vi "Defect detection.vi"(7 "File Path":path=path "C:/BeamViewImage/TESTIMAGE.png", 8 "error in":errorcluster, 10 "ROI Descriptors (Quantify 1)":T1(array[cluster])=[{"Global Rectangle"=[0, 0, 1280, 1024], "Contours"=[{"ID"=enum."External", "Type"=3, "Coordinates"=[0, 0, 1280, 1024]}]}] {"Contours"."Type" items=["No Selection", "Point", "Line", "Rectangle", "Oval", "Polygon", "Freehand Region", "Annulus", "Unused2", "Unused3", "Broken Line", "Freehand Line", "Rotated Rectangle"]}, 11 "Method (Filters 1)":T2(ring)=enum."Sobel") -> (0 "error out":errorcluster, 3 "Standard Variation":sgl)   [LabVIEW 2018]
uses:
  <vilib>/vision/NI_Vision_Development_Module.lvlib
panel:
  out "Image Out":T3(plugin-control)
  out "Results (Quantify 1)":sgl[][](array[numeric]) format="%.2f"
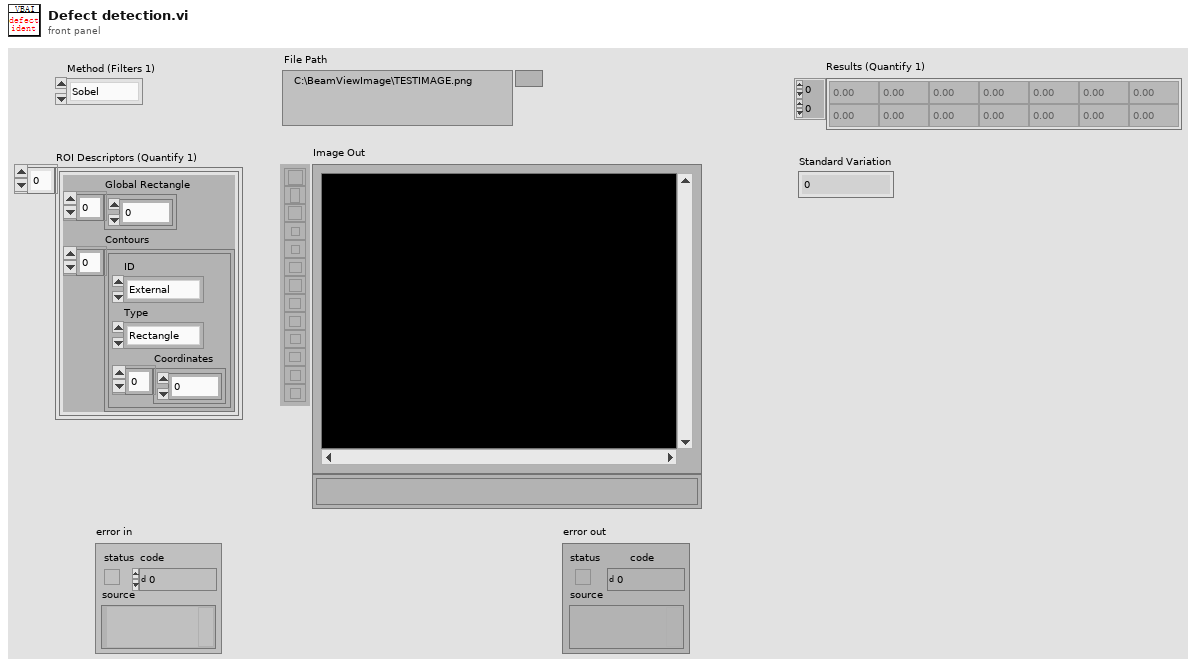
[diagram p1: front panel]
types:
  T1 = cluster{"Global Rectangle":i32[], "Contours":cluster{"ID":enum32{"External", "Internal"}, "Type":u32, "Coordinates":i32[]}[]}[]
  T2 = enum32{"Differentiation", "Gradient", "Prewitt", "Roberts", "Sigma", "Sobel"}
  T3 = typedef "IMAQ Image.ctl" = refnum<image>
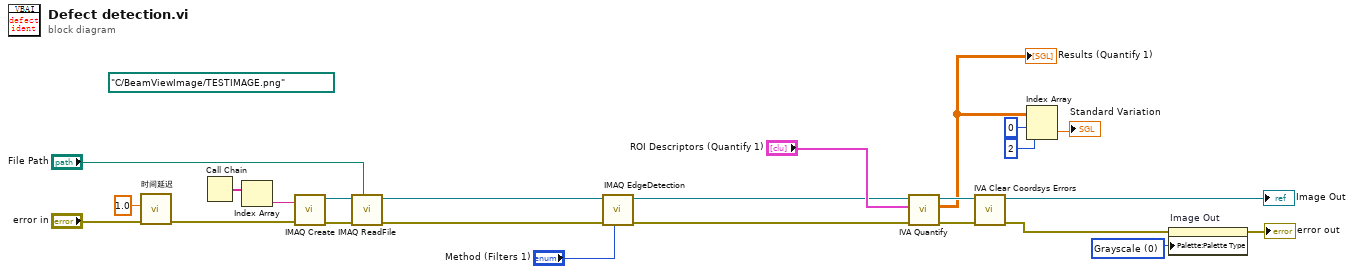
[diagram p0: block diagram]
diagram:
  (unwired) path "C:/BeamViewImage/TESTIMAGE.png" ("File Path")
  w11 = u32 0 items=["Grayscale", "Binary", "Gradient", "Rainbow", "Temperature", "User Defined", "Binary 16 Bit", "Gradient 16 Bit", "Rainbow 16 Bit", "Temperature 16 Bit", "User Defined 16 Bit"] ("Palette Type")
  n1 = call "时间延迟"("error in (no error)"="error in", "Delay Time (s)"=1.0) -> ("error out"=w2:errorcluster)  [unwired: 9 in]
  n2 = Call Chain() -> (call chain=w20:string[])
  n3 = Index Array(array=w20) -> (element=w19:string)  [unwired: 1 in]
  n4 = call "IMAQ Create"("Image Name"=w19, "error in (no error)"=w2) -> ("New Image"=w22:T3, "error out"=w21:errorcluster)  [unwired: 2 in, 1 out]
  n5 = call "IMAQ ReadFile"("File Path"="File Path", "error in (no error)"=w21, "Image"=w22) -> ("error out"=w23:errorcluster, "Image Out"=w5:T3)  [unwired: 2 in, 5 out]
  n6 = call "IMAQ EdgeDetection"("Method"="Method (Filters 1)", "error in (no error)"=w23, "Image Src"=w5) -> ("error out"=w17:errorcluster, "Image Dst Out"=w4:T3)  [unwired: 3 in, 4 out]
  n7 = call <vilib>:"IVA Quantify.vi"("error in (no error)"=w17, "ROI Descriptors"="ROI Descriptors (Quantify 1)", "Image"=w4) -> ("error out"=w15:errorcluster, "Results"=w10:sgl[][], "Image Out"=→"Image Out":T3)  [unwired: 6 out]
  "Results (Quantify 1)" <- w10
  n8 = call <vilib>:"IVA Clear Coordsys Errors.vi"("error in (no error)"=w15) -> ("error out"=w14:errorcluster)  [unwired: 10 in]
  n9 = Index Array(array=w10, index (row)=0 ("索引 (行)"), index (col)=2 ("禁用的索引 (列)")) -> (element=→"Standard Variation":sgl)
  n10 = property on="Image Out" class="ImageControl"(error in=w14, "Palette:Palette Type"=w11) -> (error out=→"error out":errorcluster)  [unwired: 1 in, 1 out]
